vi "Initiate_Web_Polling.vi"(8 "error in":errorcluster) -> (0 "error out":errorcluster)   [LabVIEW 2020]
doc: "Initiates the web polling to read the inputs from the HTML page"
uses:
  src/user_interfaces/simple_html_chat_ui/apis/WebSocket_Polling.vi
  src/user_interfaces/simple_html_chat_ui/simple_html_chat_ui.lvclass
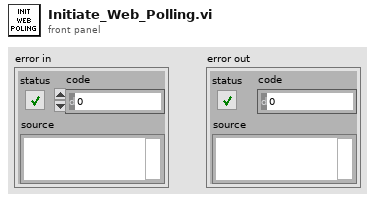
[diagram p1: front panel]
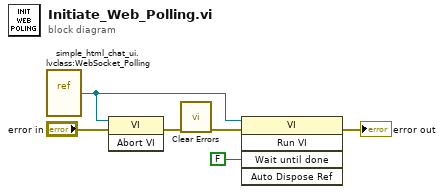
[diagram p0: block diagram]
diagram:
  n1 = vi-ref "simple_html_chat_ui.lvclass:WebSocket_Polling.vi"() -> (w6:refnum<vi>)
  n2 = invoke class="VI" method="Abort VI"(reference=w6, error in="error in") -> (error out=w2:errorcluster)  [unwired: 1 in, 2 out]
  n3 = call <vilib>:"Clear Errors.vi"("error in (no error)"=w2) -> ("error out"=w4:errorcluster)  [unwired: 5 in, 1 out]
  n4 = invoke class="VI" method="Run VI"(reference=w6, error in=w4, "Wait until done"=FALSE ("Wait Until Done")) -> (error out=→"error out":errorcluster)  [unwired: 2 in, 4 out]
